vi "resort_sinogram_data.vi"(6 "Ramp end":i32, 7 "Ramp begin":i32, 8 "Shift up and down":bool, 9 "pts per projection":i32, 10 "projections":i32=2, 11 "Input":dbl[](array[numeric])) -> (0 "Output":dbl[][](array[numeric]))   [LabVIEW 2019]
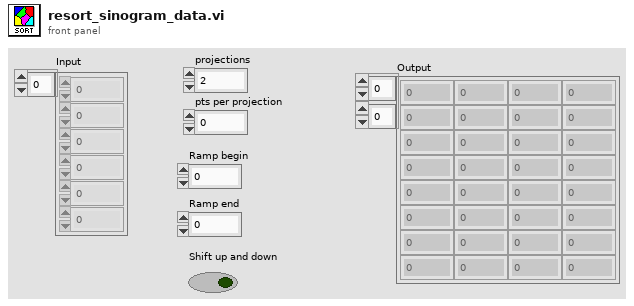
[diagram p1: front panel]
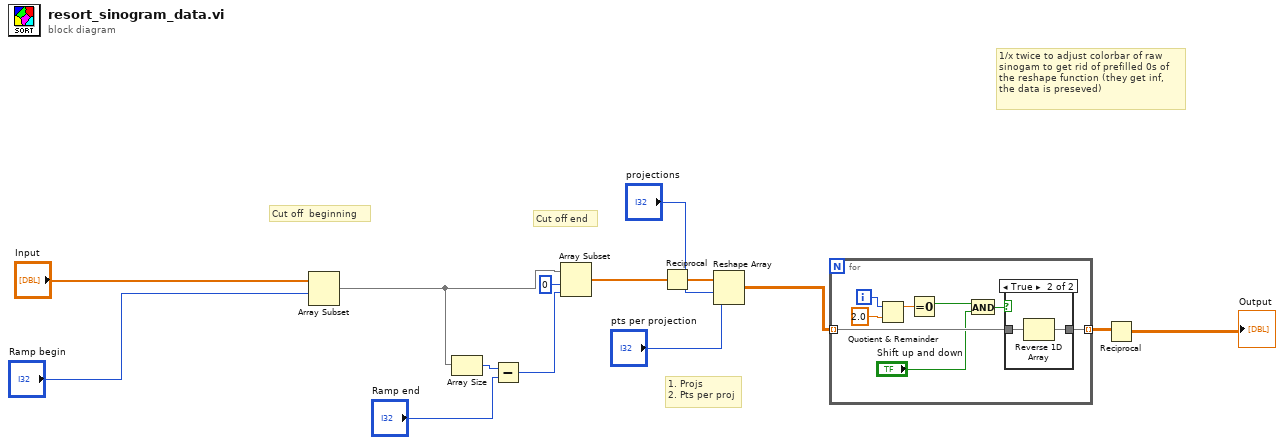
[diagram p0: block diagram]
diagram:
  # "1/x twice to adjust colorbar of raw\nsinogam to get rid of prefilled 0s of\nthe reshape function (they get inf, \nthe data is preseved)"
  # "1. Projs\n2. Pts per proj"
  # "Cut off end"
  # "Cut off  beginning"
  n1 = Array Subset(array="Input", index="Ramp begin") -> (w9:dbl[])  [unwired: 1 in]
  n2 = Array Size(array=w9) -> (size(s)=w11:i32)
  n3 = Subtract(x=w11, y="Ramp end") -> (x-y=w13:i32)
  n4 = Array Subset(array=w9, index=0, length=w13) -> (w7:dbl[])
  n5 = Reciprocal(x=w7) -> (1/x=w6:dbl[])
  n6 = Reshape Array(w6, "projections", "pts per projection") -> (w5:dbl[][])
  n7 = for {
    tunnel: w5 -> [w20] mode=indexing
    tunnel: [w19] -> w3 mode=indexing
    i -> [w18]
    n8 = Quotient & Remainder(x=w18, y=2.0) -> (x-y*floor(x/y)=w21:dbl)  [unwired: 1 out]
    n9 = Equal To 0?(x=w21) -> (x = 0?=w16:bool)
    n10 = And(x=w16, y="Shift up and down") -> (x .and. y?=w17:bool)
    n11 = case shown="True" w17 {
      tunnel: w20 -> [w23 w25]
      tunnel: [w23 w24] -> w19
      frame False {
      }
      frame True {
        n12 = Reverse 1D Array(array=w25) -> (reversed array=w24:dbl[])
      }
    }
  }
  n13 = Reciprocal(x=w3) -> (1/x=→"Output":dbl[][])
